vi "Solve2.vi"(8 "Error In":errorcluster, 11 "object in":refnum<class "2021_15.lvclass">) -> (0 "Error Out":errorcluster, 2 "Result":u64, 3 "object out":refnum<class "2021_15.lvclass">)   [LabVIEW 2020, in "2021_15.lvclass"]
uses:
  2021_15.lvclass
  2021_15.lvclass/2021_15.ctl
panel:
  out "Array 2":i32[][](array[numeric])
  out "Array":i32[][](array[numeric])
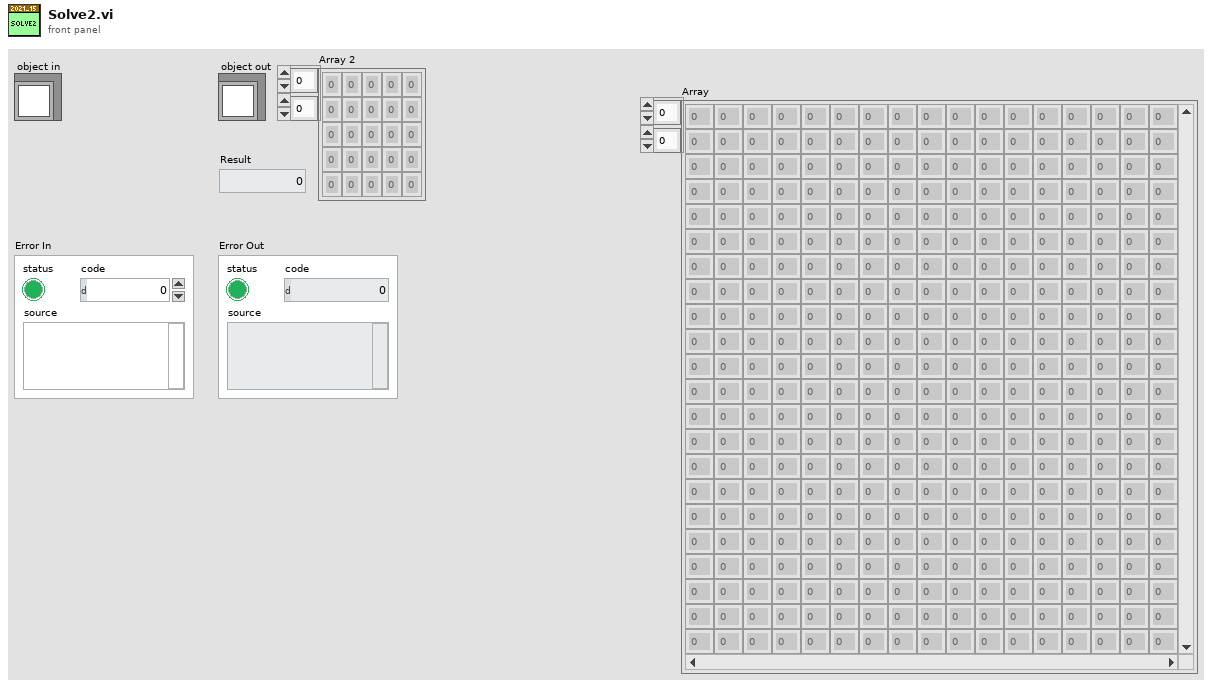
[diagram p1: front panel]
types:
  T1 = typedef "NI_Matrix.lvlib/RealMatrix.ctl" = dbl[][]
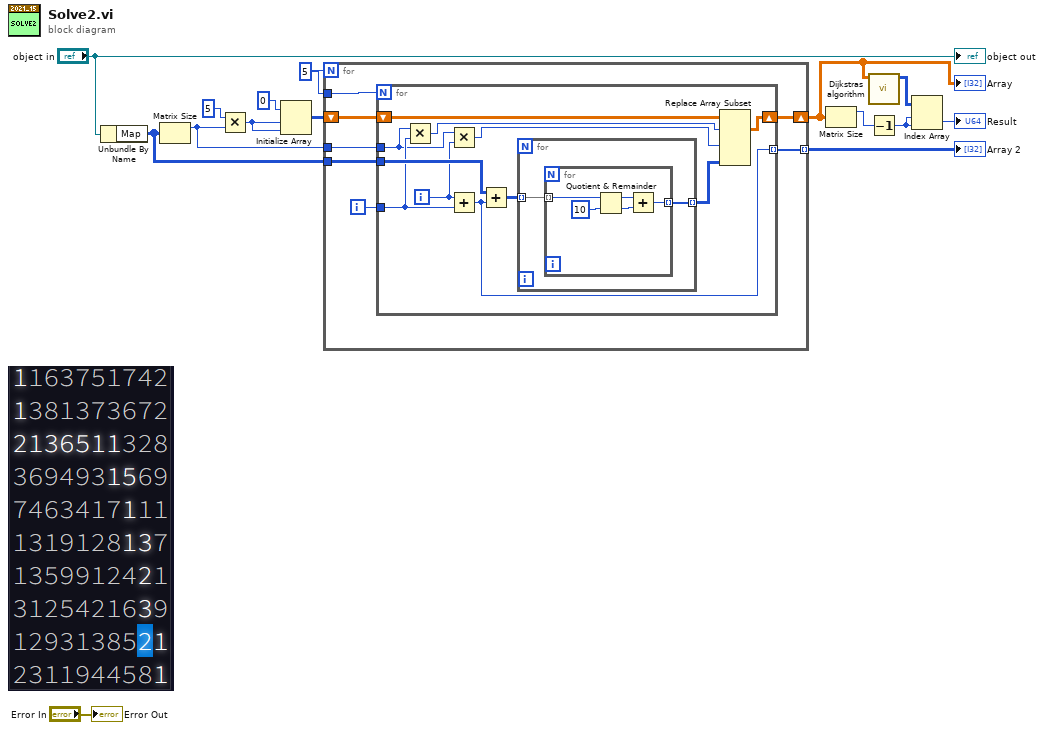
[diagram p0: block diagram]
diagram:
  w8 = 5
  n1 = Unbundle By Name("object in") -> ("Map"=w13:u8[][])
  n2 = Matrix Size(0:w13) -> (1:w2:i32)  [unwired: 1 out]
  n3 = Multiply(x=5, y=w2) -> (x*y=w6:i32)
  n4 = Initialize Array(0 ("x"), w6, w6) -> (w3:i32[][])
  n5 = for {
    N: w8 -> [_]
    tunnel: w8 -> [w22]
    tunnel: [w20] -> w4 mode=indexing
    tunnel: w13 -> [w19]
    shift-right: [w17] -> w1
    shift-left: w3 -> [w18]
    tunnel: w2 -> [w16]
    i -> [w21]
    n6 = for {
      N: w22 -> [_]
      tunnel: w21 -> [w29]
      tunnel: [w32] -> w20 mode=indexing
      tunnel: w19 -> [w33]
      shift-right: [w30] -> w17
      shift-left: w18 -> [w31]
      tunnel: w16 -> [w26]
      i -> [w27]
      n7 = Multiply(x=w26, y=w29) -> (x*y=w28:i32)
      n8 = Multiply(x=w26, y=w27) -> (x*y=w25:i32)
      n9 = Add(x=w27, y=w29) -> (x+y=w32:i32)
      n10 = Add(x=w33, y=w32) -> (x+y=w24:i32[][])
      n11 = for {
        tunnel: w24 -> [w35] mode=indexing
        tunnel: [w34] -> w23 mode=indexing
        n12 = for {
          tunnel: w35 -> [w40] mode=indexing
          tunnel: [w36] -> w34 mode=indexing
          n13 = Quotient & Remainder(x=w40, y=10) -> (x-y*floor(x/y)=w37:i32, floor(x/y)=w38:i32)
          n14 = Add(x=w37, y=w38) -> (x+y=w36:i32)
        }
      }
      n15 = Replace Array Subset(array=w31, new element=w23, index (dim 0)=w28, index (dim 2)=w25) -> (w30:T1)  [unwired: 2 in]
    }
  }
  "Array" <- w1
  "Array 2" <- w4
  n16 = Matrix Size(0:w1) -> (1:w10:i32)  [unwired: 1 out]
  n17 = call "Dijkstras algorithm.vi"("Map"=w1) -> ("Array"=w11:i32[][])  [unwired: 10 in]
  n18 = Decrement(x=w10) -> (x-1=w9:i32)
  n19 = Index Array(array=w11, index (row)=w9, index (col)=w9) -> (element=→"Result":i32)
  "Error Out" <- "Error In"
  "object out" <- "object in"
